vi "Do Update UI Event.vi"(7 "MulticolumnListbox in":refnum<vi>, 8 "error in":errorcluster, 11 "Update UI Data":variant) -> (0 "error out":errorcluster, 2 "Assert VI UID Array":i32[](array[numeric]))   [LabVIEW 2016, in "Assert API Components.lvlib" / "Assert Display.lvlib" / "Main Display.lvlib" / "Main Display.lvclass"]
uses:
  Main Display.lvclass
  Components/Display Data.ctl
  Display Colours.ctl
  Main Display.lvlib
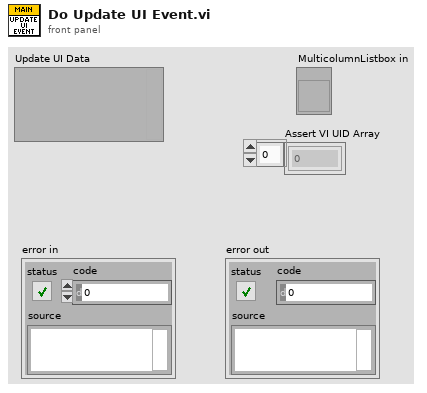
[diagram p1: front panel]
types:
  T1 = typedef "Assert API Components.lvlib/Assert Display.lvlib/Main Display.lvlib/Display Data.ctl" = cluster{"ItemNames":string[][], "Pass Fail Status":bool[], "Display Colours":T2, "Assert VI UID Array":i32[]}
  T2 = typedef "Assert API Components.lvlib/Assert Display.lvlib/Main Display.lvlib/Display Colours.ctl" = cluster{"Enable Colours":bool, "Passed Colour":u32, "Failed Colour":u32}
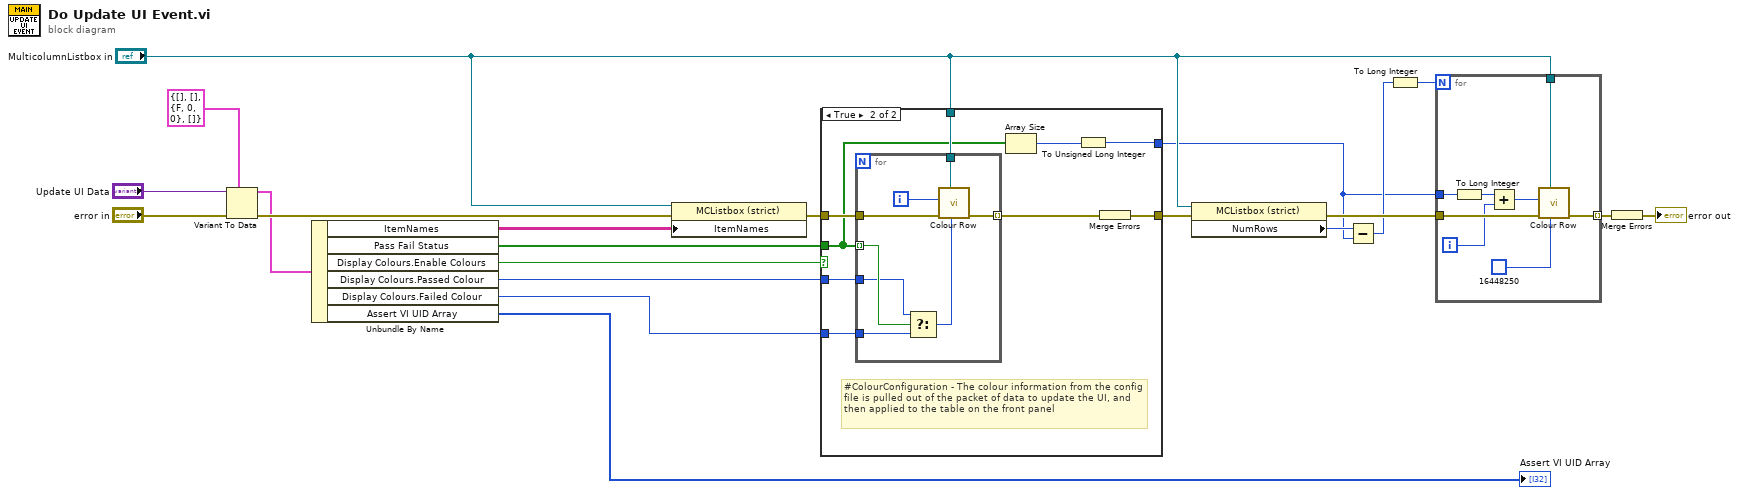
[diagram p0: block diagram]
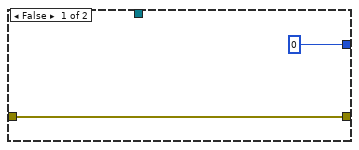
[diagram p2: hidden frame]
diagram:
  n1 = Variant To Data(error in="error in", type=T1 {"ItemNames"=[], "Pass Fail Status"=[], "Display Colours"={"Enable Colours"=FALSE, "Passed Colour"=0, "Failed Colour"=0}, "Assert VI UID Array"=[]}, Variant="Update UI Data") -> (data=w16:T1, error out=w20:errorcluster)
  n2 = Unbundle By Name(w16) -> ("ItemNames"=w15:string[][], "Pass Fail Status"=w14:bool[], "Display Colours.Enable Colours"=w13:bool, "Display Colours.Passed Colour"=w12:u32, "Display Colours.Failed Colour"=w11:u32, "Assert VI UID Array"=→"Assert VI UID Array":i32[])
  n3 = property on="Property Node" class="MCListbox (strict)"(reference="MulticolumnListbox in", error in=w20, "ItemNames"=w15) -> (error out=w21:errorcluster)  [unwired: 1 out]
  n4 = case shown="True" w13 {
    tunnel: w21 -> [w23 w30]
    tunnel: [w23 w27] -> w10
    tunnel: w14 -> [_ w26]
    tunnel: w12 -> [_ w32]
    tunnel: w11 -> [_ w31]
    tunnel: "MulticolumnListbox in" -> [_ w29]
    tunnel: [u32 0 w24] -> w1
    frame False {
    }
    frame True {
      # "#ColourConfiguration - The colour information from the config file is pulled out of the packet of data to update the UI, and then applied to the table on the front panel"
      n5 = for {
        tunnel: w26 -> [w40] mode=indexing
        tunnel: w32 -> [w39]
        tunnel: w31 -> [w38]
        tunnel: w29 -> [w33]
        tunnel: w30 -> [w37]
        tunnel: [w36] -> w28 mode=indexing
        i -> [w35]
        n6 = Select(t=w39, s=w40, f=w38) -> (s? t:f=w34:u32)
        n7 = call "Colour Row.vi"("Row Colour"=w34, "MulticolumnListbox in"=w33, "error in (no error)"=w37, "Row Number"=w35) -> ("error out"=w36:errorcluster)  [unwired: 7 in]
      }
      n8 = Array Size(array=w26) -> (size(s)=w25:i32)
      n9 = To Unsigned Long Integer(number=w25) -> (unsigned 32bit integer=w24:u32)
      n10 = Merge Errors(w28) -> (w27:errorcluster)
    }
  }
  n11 = property class="MCListbox (strict)"(reference="MulticolumnListbox in", error in=w10) -> (error out=w7:errorcluster, "NumRows"=w4:u32)  [unwired: 1 out]
  n12 = Subtract(x=w4, y=w1) -> (x-y=w3:u32)
  n13 = To Long Integer(number=w3) -> (32bit integer=w2:i32)
  n14 = for {
    N: w2 -> [_]
    tunnel: w7 -> [w48]
    tunnel: [w47] -> w9 mode=indexing
    tunnel: "MulticolumnListbox in" -> [w46]
    tunnel: w1 -> [w43]
    i -> [w44]
    n15 = To Long Integer(number=w43) -> (32bit integer=w41:i32)
    n16 = Add(x=w41, y=w44) -> (x+y=w42:i32)
    n17 = call "Colour Row.vi"("Row Colour"=u32 16448250, "MulticolumnListbox in"=w46, "error in (no error)"=w48, "Row Number"=w42) -> ("error out"=w47:errorcluster)  [unwired: 7 in]
  }
  n18 = Merge Errors(w9) -> (→"error out":errorcluster)
